vi "Unflatten.vi"(8 "error in (no error)":errorcluster, 11 "Wavelength Digikröm in":refnum<class "Wavelength Digikröm.lvclass">) -> (0 "error out":errorcluster, 3 "Wavelength Digikröm out":refnum<class "Wavelength Digikröm.lvclass">)   [LabVIEW 2017, in "Wavelength Digikröm.lvclass"]
uses:
  Global/File Locations.vi
  Scanner/Scanner.lvclass
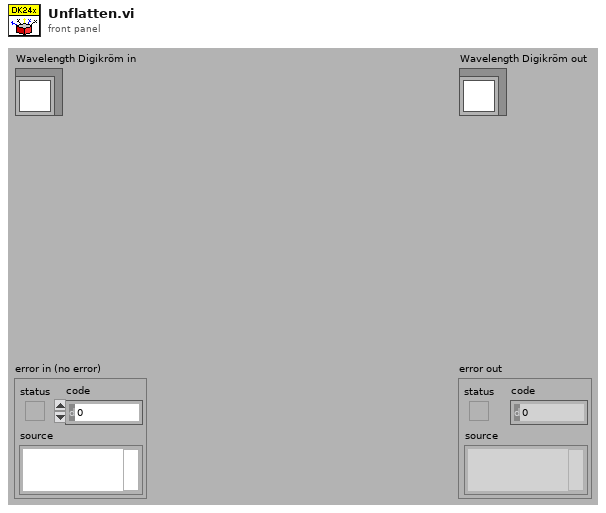
[diagram p1: front panel]
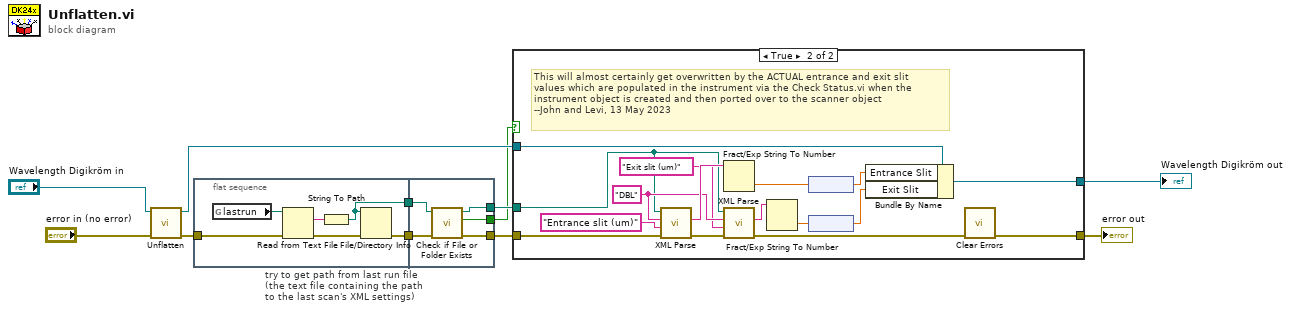
[diagram p0: block diagram]
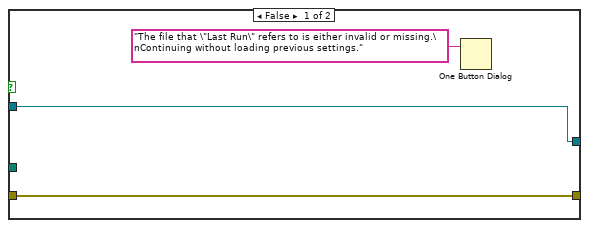
[diagram p2: hidden frame]
diagram:
  n1 = call-parent "Unflatten.vi"("error in (no error)"="error in (no error)", "Scanner in"="Wavelength Digikröm in") -> ("error out"=w7:errorcluster, "Scanner out"=w11:refnum<class "Wavelength Digikröm.lvclass">)  [unwired: 8 in]
  n2 = flat-sequence "try to get path from last run file\n(the text file containing the path\nto the last scan's XML settings)" {
    tunnel: w7 -> [w12]
    tunnel: [w17] -> w3
    tunnel: [w13] -> w2
    tunnel: [w21] -> w6
    tunnel: [w22] -> w5
    tunnel: w3 -> [w19]
    tunnel: w2 -> [w20]
    tunnel: [w18] -> w1
    frame #0 {
      n3 = global read "File Locations.vi" "lastrun"() -> (w15:path)
      n4 = Read from Text File(file (use dialog)=w15, error in=w12) -> (text=w16:string, error out=w14:errorcluster)  [unwired: 4 out]
      n5 = String To Path(string=w16) -> (path=w17:path)
      n6 = File/Directory Info(path=w17, error in=w14) -> (error out=w13:errorcluster)  [unwired: 6 out]
    }
    frame #1 {
      n7 = call <vilib>:"Check if File or Folder Exists.vi"("error in (no error)"=w20, "path"=w19) -> ("error out"=w21:errorcluster, "file or folder exists?"=w18:bool, "dup path"=w22:path)  [unwired: 7 in]
    }
  }
  n8 = case shown="True" w1 {
    tunnel: w11 -> [w23 w41]
    tunnel: [w23 w40] -> w8
    tunnel: w6 -> [w24 w39]
    tunnel: w5 -> [_ w32]
    tunnel: [w24 w37] -> w4
    frame False {
      n9 = One Button Dialog(message="The file that \"Last Run\" refers to is either invalid or missing.\nContinuing without loading previous settings.") -> ()  [unwired: 1 in, 1 out]
    }
    frame True {
      w33 = "DBL"
      # "This will almost certainly get overwritten by the ACTUAL entrance and exit slit \nvalues which are populated in the instrument via the Check Status.vi when the \ninstrument object is created and then ported over to the scanner object\n--John and Levi, 13 May 2023"
      n10 = call "XML Parse.vi"("error in (no error)"=w39, "Name String"="Entrance slit (um)", "Type String"=w33, "Path"=w32) -> ("error out"=w30:errorcluster, "String Out"=w36:string)  [unwired: 6 in]
      n11 = Fract/Exp String To Number(string=w36) -> (number=w34:dbl)  [unwired: 3 in, 1 out]
      n12 = call "XML Parse.vi"("error in (no error)"=w30, "Name String"="Exit slit (um)", "Type String"=w33, "Path"=w32) -> ("error out"=w26:errorcluster, "String Out"=w29:string)  [unwired: 6 in]
      n13 = Fract/Exp String To Number(string=w29) -> (number=w28:dbl)  [unwired: 3 in, 1 out]
      n14 = node(w34) -> (w35:dbl[unit])
      n15 = node(w28) -> (w27:dbl[unit])
      n16 = Bundle By Name(cluster=w41, "Entrance Slit"=w35, "Exit Slit"=w27) -> (w40:refnum<class "Wavelength Digikröm.lvclass">)
      n17 = call <vilib>:"Clear Errors.vi"("error in (no error)"=w26) -> ("error out"=w37:errorcluster)  [unwired: 5 in, 1 out]
    }
  }
  "error out" <- w4
  "Wavelength Digikröm out" <- w8
